vi "generatore_quadra_0_1.vi"(0 "f0 (frequenza base) [Hz]":dbl min=0.0, 1 "Ap (ampiezza di picco)":dbl min=0.0, 2 "Tc (periodo di campionamento) [s]":dbl min=0.0, 3 "Ta (tempo di analisi) [s]":dbl min=0.0, 5 "Phi (fase iniziale) [rad]":dbl, 8 "DC Offset":dbl) -> (7 "Waveform Graph":waveform(dbl)(graph))   [LabVIEW 2009]
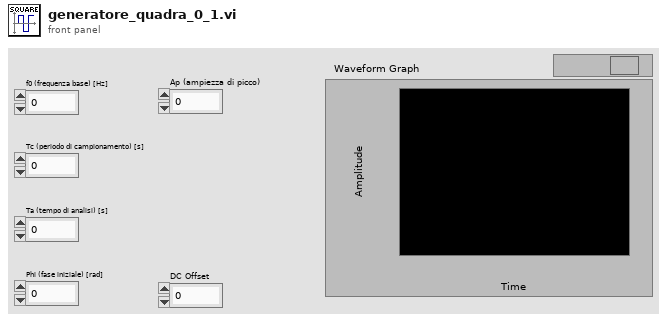
[diagram p1: front panel]
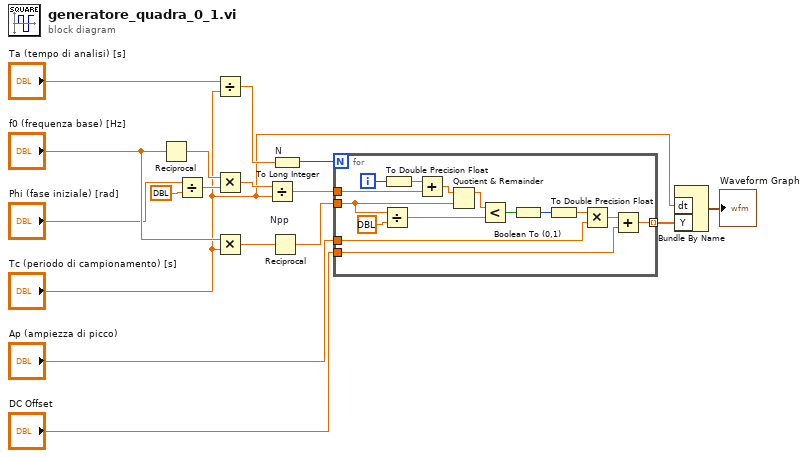
[diagram p0: block diagram]
diagram:
  n1 = Reciprocal(x="f0 (frequenza base) [Hz]") -> (1/x=w5:dbl)
  n2 = Divide(x="Phi (fase iniziale) [rad]", y=dbl ?) -> (x/y=w6:dbl)
  n3 = Divide(x="Ta (tempo di analisi) [s]", y="Tc (periodo di campionamento) [s]") -> (x/y=w12:dbl)
  n4 = Multiply(x=w5, y=w6) -> (x*y=w4:dbl)
  n5 = Multiply(x="f0 (frequenza base) [Hz]", y="Tc (periodo di campionamento) [s]") -> (x*y=w16:dbl)
  n6 = Divide(x=w4, y="Tc (periodo di campionamento) [s]") -> (x/y=w2:dbl)
  n7 = Reciprocal "Npp"(x=w16) -> (1/x=w17:dbl)
  n8 = To Long Integer "N"(number=w12) -> (32bit integer=w13:i32)
  n9 = for {
    N: w13 -> [_]
    tunnel: "DC Offset" -> [w32]
    tunnel: "Ap (ampiezza di picco)" -> [w19]
    tunnel: [w31] -> w10 mode=indexing
    tunnel: w17 -> [w30]
    tunnel: w2 -> [w20]
    i -> [w29]
    n10 = Divide(x=w30, y=dbl ?) -> (x/y=w25:dbl)
    n11 = To Double Precision Float(number=w29) -> (double precision float=w28:dbl)
    n12 = Add(x=w28, y=w20) -> (x+y=w27:dbl)
    n13 = Quotient & Remainder(x=w27, y=w30) -> (x-y*floor(x/y)=w26:dbl)  [unwired: 1 out]
    n14 = Less?(x=w26, y=w25) -> (x < y?=w24:bool)
    n15 = Boolean To (0,1)(Boolean=w24) -> (0, 1=w23:i16)
    n16 = To Double Precision Float(number=w23) -> (double precision float=w22:dbl)
    n17 = Multiply(x=w22, y=w19) -> (x*y=w18:dbl)
    n18 = Add(x=w18, y=w32) -> (x+y=w31:dbl)
  }
  n19 = Bundle By Name("dt"="Tc (periodo di campionamento) [s]", "Y"=w10) -> (→"Waveform Graph":waveform(dbl))  [unwired: 1 in]
